vi "Monitor.vi"(10 "Information":refnum<vi>, 11 "Port 2":refnum<vi>) -> (0 "Process":T1, 2 "Information":refnum<vi>, 3 "reference out":refnum<vi>)   [LabVIEW 2013]
uses:
  Control/SystemProcess.ctl
  Control/Buffer.vi
  <vilib>/DAQmx/create/channels.llb/DAQmx Create Channel (DI-Digital Input).vi
  <vilib>/DAQmx/read.llb/DAQmx Read (Digital 1D Bool 1Chan 1Samp).vi
panel:
  out "Array":bool[](array[boolean])
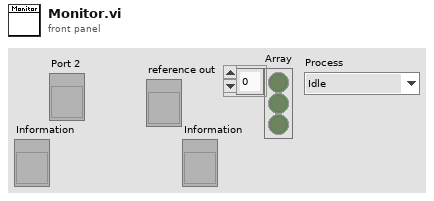
[diagram p1: front panel]
types:
  T1 = typedef "SystemProcess.ctl" = enum16{"Idle", "SystemInit", "SpecialEvent", "Barcode(SN)", "TestInitialize", "Test", "Stop", "SaveTestData", "Exit"}
  T2 = typedef "Port.ctl" = cluster{"Multimeter":refnum<visa-resource-name>, "ACsource ":refnum<visa-resource-name>, "GEA":refnum<visa-resource-name>, "LEDanalizer":refnum<visa-resource-name>, "AutoScan":refnum<visa-resource-name>, "lines":tag, "MabeCOM":refnum<visa-resource-name>}
  T3 = typedef "StatusInformation.ctl" = cluster{"FileName:":string, "Barcode(S/N):":string, "TestStep:":string, "TestTime:":string, "Station:":string, "Model:":string, "Line:":string, "Status:":string, "Series:":string, "Reserve:":string}
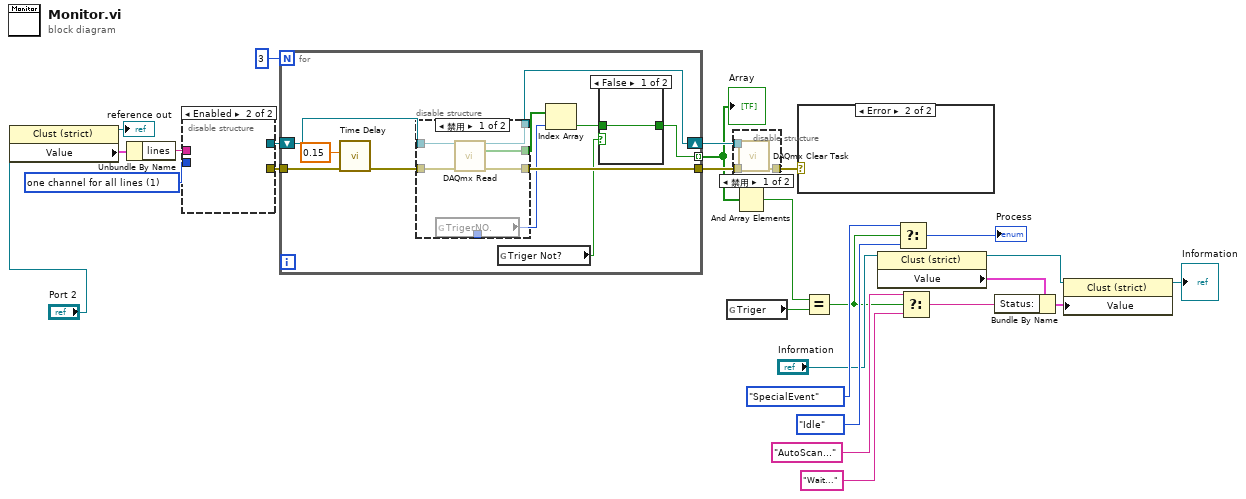
[diagram p0: block diagram]
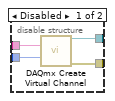
[diagram p3: hidden frame]
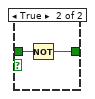
[diagram p6: hidden frame]
diagram:
  w26 = 1 items=["one channel for each line", "one channel for all lines"] ("line grouping")
  n1 = property class="Clust (strict)"(reference="Port 2") -> (reference out=→"reference out":refnum<vi>, "Value"=w16:T2)  [unwired: 1 in, 1 out]
  n2 = Unbundle By Name(w16) -> ("lines"=w15:tag)
  n3 = disable-structure shown="Enabled" {
    disable-tunnel: w26 -> [w30 _]
    disable-tunnel: [w29 _] -> w24
    disable-tunnel: [w28 _] -> w22
    disable-tunnel: w15 -> [w27 _]
    frame Disabled {
      n4 = call-poly <vilib>:"DAQmx Create Virtual Channel.vi"("lines"=w27, "line grouping"=w30) -> ("task out"=w29:refnum<k21>, "error out"=w28:errorcluster)  [unwired: 12 in]
    }
    frame Enabled {
    }
  }
  n5 = for {
    N: 3 -> [_]
    shift-right: [w38] -> w23
    shift-left: w24 -> [w39]
    tunnel: w22 -> [w37]
    tunnel: [w33] -> w20 mode=indexing
    tunnel: [w36] -> w21
    n6 = call "Time Delay"("error in (no error)"=w37, "Delay Time (s)"=0.15) -> ("error out"=w40:errorcluster)  [unwired: 9 in]
    n7 = disable-structure shown="禁用" {
      disable-tunnel: w40 -> [w47 _]
      disable-tunnel: w39 -> [w46 _]
      disable-tunnel: [w45 _] -> w38
      disable-tunnel: [w44 _] -> w36
      disable-tunnel: [w43 _] -> w35
      disable-tunnel: [w42 _] -> w31
      frame Disabled {
        n8 = global read "Buffer.vi" "TrigerNO."() -> (w42:i32)
        n9 = call-poly <vilib>:"DAQmx Read.vi"("task/channels in"=w46, "error in"=w47) -> ("task out"=w45:refnum<k21>, "data"=w43:bool[], "error out"=w44:errorcluster)  [unwired: 11 in]
      }
      frame Enabled {
      }
    }
    n10 = global read "Buffer.vi" "Triger Not?"() -> (w32:bool)
    n11 = Index Array(array=w35, index=w31) -> (element=w34:bool)
    n12 = case shown="False" w32 {
      tunnel: w34 -> [w48 w50]
      tunnel: [w48 w49] -> w33
      frame False {
      }
      frame True {
        n13 = Not(x=w50) -> (.not. x?=w49:bool)
      }
    }
  }
  "Array" <- w20
  n14 = global read "Buffer.vi" "Triger"() -> (w5:bool)
  n15 = disable-structure shown="禁用" {
    disable-tunnel: w23 -> [w53 _]
    disable-tunnel: w21 -> [w52 _]
    disable-tunnel: [w51 _] -> w6
    frame Disabled {
      n16 = call <vilib>:"DAQmx Clear Task.vi"("task in"=w53, "error in"=w52) -> ("error out"=w51:errorcluster)  [unwired: 13 in]
    }
    frame Enabled {
    }
  }
  n17 = And Array Elements(Boolean array=w20) -> (logical AND=w4:bool)
  n18 = case shown="Error" w6 {
    frame No Error {
    }
    frame Error {
    }
  }
  n19 = Equal?(x=w4, y=w5) -> (x = y?=w3:bool)
  n20 = property class="Clust (strict)"(reference="Information") -> (reference out=w11:refnum<vi>, "Value"=w10:T3)  [unwired: 1 in, 1 out]
  n21 = Select(t=SystemProcess."SpecialEvent", s=w3, f=SystemProcess."Idle" ("MainProcess")) -> (s? t:f=→"Process":T1)
  n22 = Select(t="AutoScan...", s=w3, f="Wait...") -> (s? t:f=w9:string)
  n23 = Bundle By Name(cluster=w10, "Status:"=w9) -> (w8:T3)
  n24 = property class="Clust (strict)"(reference=w11, "Value"=w8) -> (reference out=→"Information":refnum<vi>)  [unwired: 1 in, 1 out]
